vi "Main.vi"(11 "Module Admin":refnum<class "Delacor_lib_QMH_Module Admin.lvclass">) -> ()   [LabVIEW 2021, in "AS-Configuration.lvlib"]
doc: "This template is based off of the Queued Message Handler design pattern and the Queued Message Handler project template that ships with LabVIEW.\n\nThe main difference is that the queue is private to this module and communication between modules is performed via Broadcast and Request events.\n\nRequest events are wrapped in public API methods and are handled in the Event Handling Loop (EHL) of this VI. Any module can register for Broadcast events sent by this module. The EHL generates messages based on user interface actions.\n\nThe Message Handling Loop (MHL) processes messages generated by the EHL, or by other messages. The messages are string values, so new messages can be added easily to the Message Cases case structure in the MHL. Each message cluster can also provide an optional value for Message Data, which is a variant that can be converted to whatever message-specific data is required.\n_____\nBased on DQMH Project Template 7.0.1.1316."
uses:
  AS-Configuration.lvlib
  <vilib>/Delacor/Delacor QMH/Libraries/Module Admin_class/Delacor_lib_QMH_Module Admin.lvclass
  Module Data--cluster.ctl
  Configuration/DO Channel's.ctl
  <vilib>/Wovalab/Utilities/Helper Loop Periodic Timing/Helper Loop Periodic Timing.lvclass/Helper Loop Periodic Timing.ctl
  <vilib>/Delacor/Delacor QMH/Libraries/Message Queue_class/Delacor_lib_QMH_Message Queue.lvclass/Delacor_lib_QMH_Message Queue.ctl
  Stop Argument--cluster.ctl
  <vilib>/Delacor/Delacor QMH/Libraries/Module Admin_class/Delacor_lib_QMH_Module Admin.lvclass/Delacor_lib_QMH_Module Admin.ctl
  <vilib>/Utility/miscctls.llb/LVPointTypeDef.ctl
  Host-Control's/DTT Test folder Name's.ctl
  <vilib>/Delacor/Delacor QMH/Libraries/Message Queue_class/Delacor_lib_QMH_Enqueue Message (Single).vi
  <vilib>/Delacor/Delacor QMH/Libraries/Module Admin_class/Delacor_lib_QMH_Get External Launch.vi
  <vilib>/Wovalab/Utilities/Helper Loop Periodic Timing/U32 Max Value--constant.vi
  <vilib>/Wovalab/Utilities/Helper Loop Periodic Timing/Update Last Execution Time.vi
  <vilib>/Utility/traverseref.llb/TRef Get All FP References.vi
  <vilib>/Utility/traverseref.llb/Get GObject Label.vi
  <vilib>/Utility/xml.llb/Read From XML File.vi
  <vilib>/Utility/xml.llb/Read From XML File(string).vi
  <vilib>/Utility/xml.llb/Write to XML File.vi
  <vilib>/Utility/xml.llb/Write to XML File(string).vi
  <vilib>/Wovalab/Utilities/Helper Loop Periodic Timing/Helper Loop Periodic Timing.lvclass
  <vilib>/Delacor/Delacor QMH/Libraries/Message Queue_class/Delacor_lib_QMH_Message Queue.lvclass
  Main-Module/Host Main.lvlib
  <userlib>/_OpenG.lib/appcontrol/appcontrol.llb/openg_application_control.lvlib
  Configuration/Configuration.lvlib
panel:
  out "Refnum OK?":bool
  out "Given File Name":string
  out "Hw Config File":string caption="Hardware Config File Name"
  in  "New":bool
  in  "Open":bool
  in  "Save":bool
  in  "Table":T1(array[cluster]) {"End Time (S)" min=0.0 max=60.0 step=1.0; "Start Time" min=0.0 max=60.0 step=1.0}
  out "AS-File Name":string caption="Auto-Sequence File Name"
  out "error out":errorcluster
  out "Status":string
  in  "Simulate MHL Error":bool
  in  "Simulate EHL Error":bool
  # "IIT M Drop Tower Test System"
  # "Auto-Sequence Configuration"
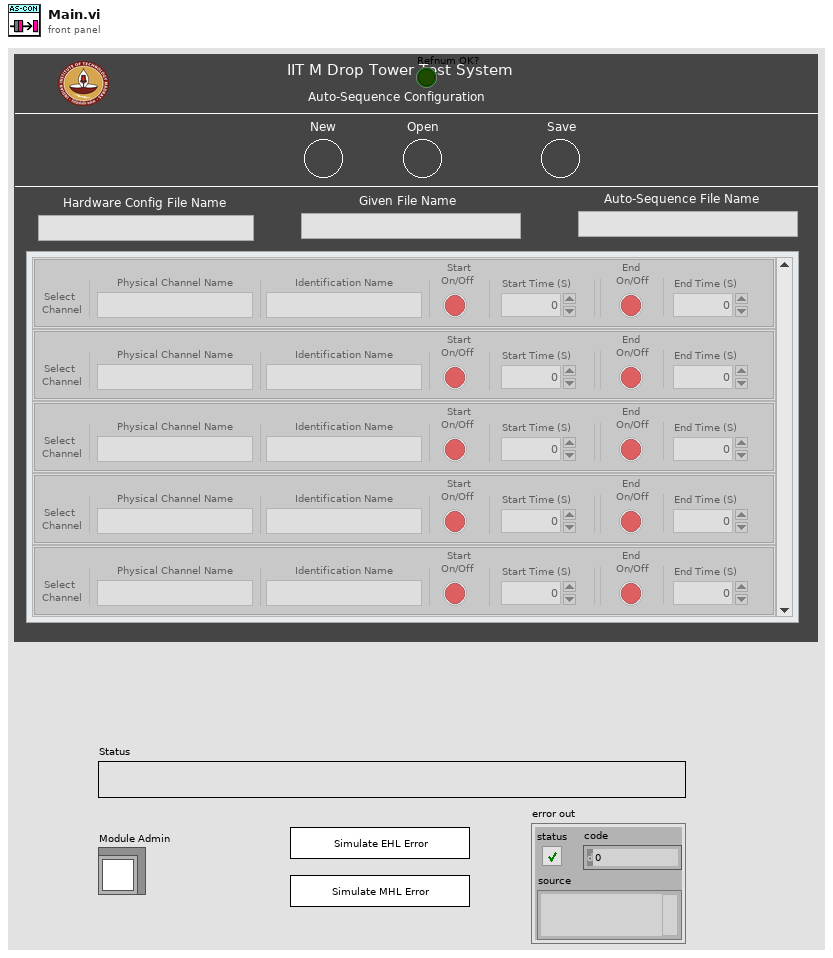
[diagram p1: front panel]
types:
  T1 = cluster{"Select Channel":bool, "Physical Channel Name":string, "Identification Name":string, "  Start\nOn/Off":bool, "Start Time":dbl, "  End\nOn/Off":bool, "End Time (S)":dbl}[]
  T2 = typedef "AS-Configuration.lvlib/Request Events--cluster.ctl" = cluster{"Stop Module":refnum<user-event>, "Show Panel":refnum<user-event>, "Hide Panel":refnum<user-event>, "Get Module Execution Status":refnum<user-event>, "Show Diagram":refnum<user-event>}
  T3 = typedef "AS-Configuration.lvlib/Module Data--cluster.ctl" = cluster{"Status":string, "DO-DI Channel's":T4, "This VI":refnum<vi>, "HW Config File Name":string, "Given File Name":string, "AS-Folder Path":path, "GUI Info's":cluster{"All Object Ref":refnum<vi>[], "All Object Label":string[]}}
  T4 = typedef "Configuration.lvlib/DO Channel's.ctl" = cluster{"Channel Name":string, "Identification Name":string, "Data":u8[], "Enabled?":bool}[]
  T5 = enum32{"invalid lock state", "Not Locked", "Locked (No Password)", "Password-protected"}
  T6 = typedef "AS-Configuration.lvlib/Stop Argument--cluster.ctl" = cluster{"Origin":string, "Exit via Stop Module Req?":bool, "Wait for Module to stop?":bool}
  T7 = typedef "LVPointTypeDef.ctl" = cluster{"Horizontal":i16, "Vertical":i16}
  T8 = enum32{"Invalid", "Standard", "Closed", "Hidden", "Minimized", "Maximized"}
  T9 = typedef "DTT Test folder Name's.ctl" = enum16{"Event Log", "Auto Sequence Configuration", "Channel Configuration's"}
  T10 = cluster{"Select Channel":bool, "Physical Channel Name":string, "Identification Name":string, "  Start\nOn/Off":bool, "Start Time":dbl, "  End\nOn/Off":bool, "End Time (S)":dbl}
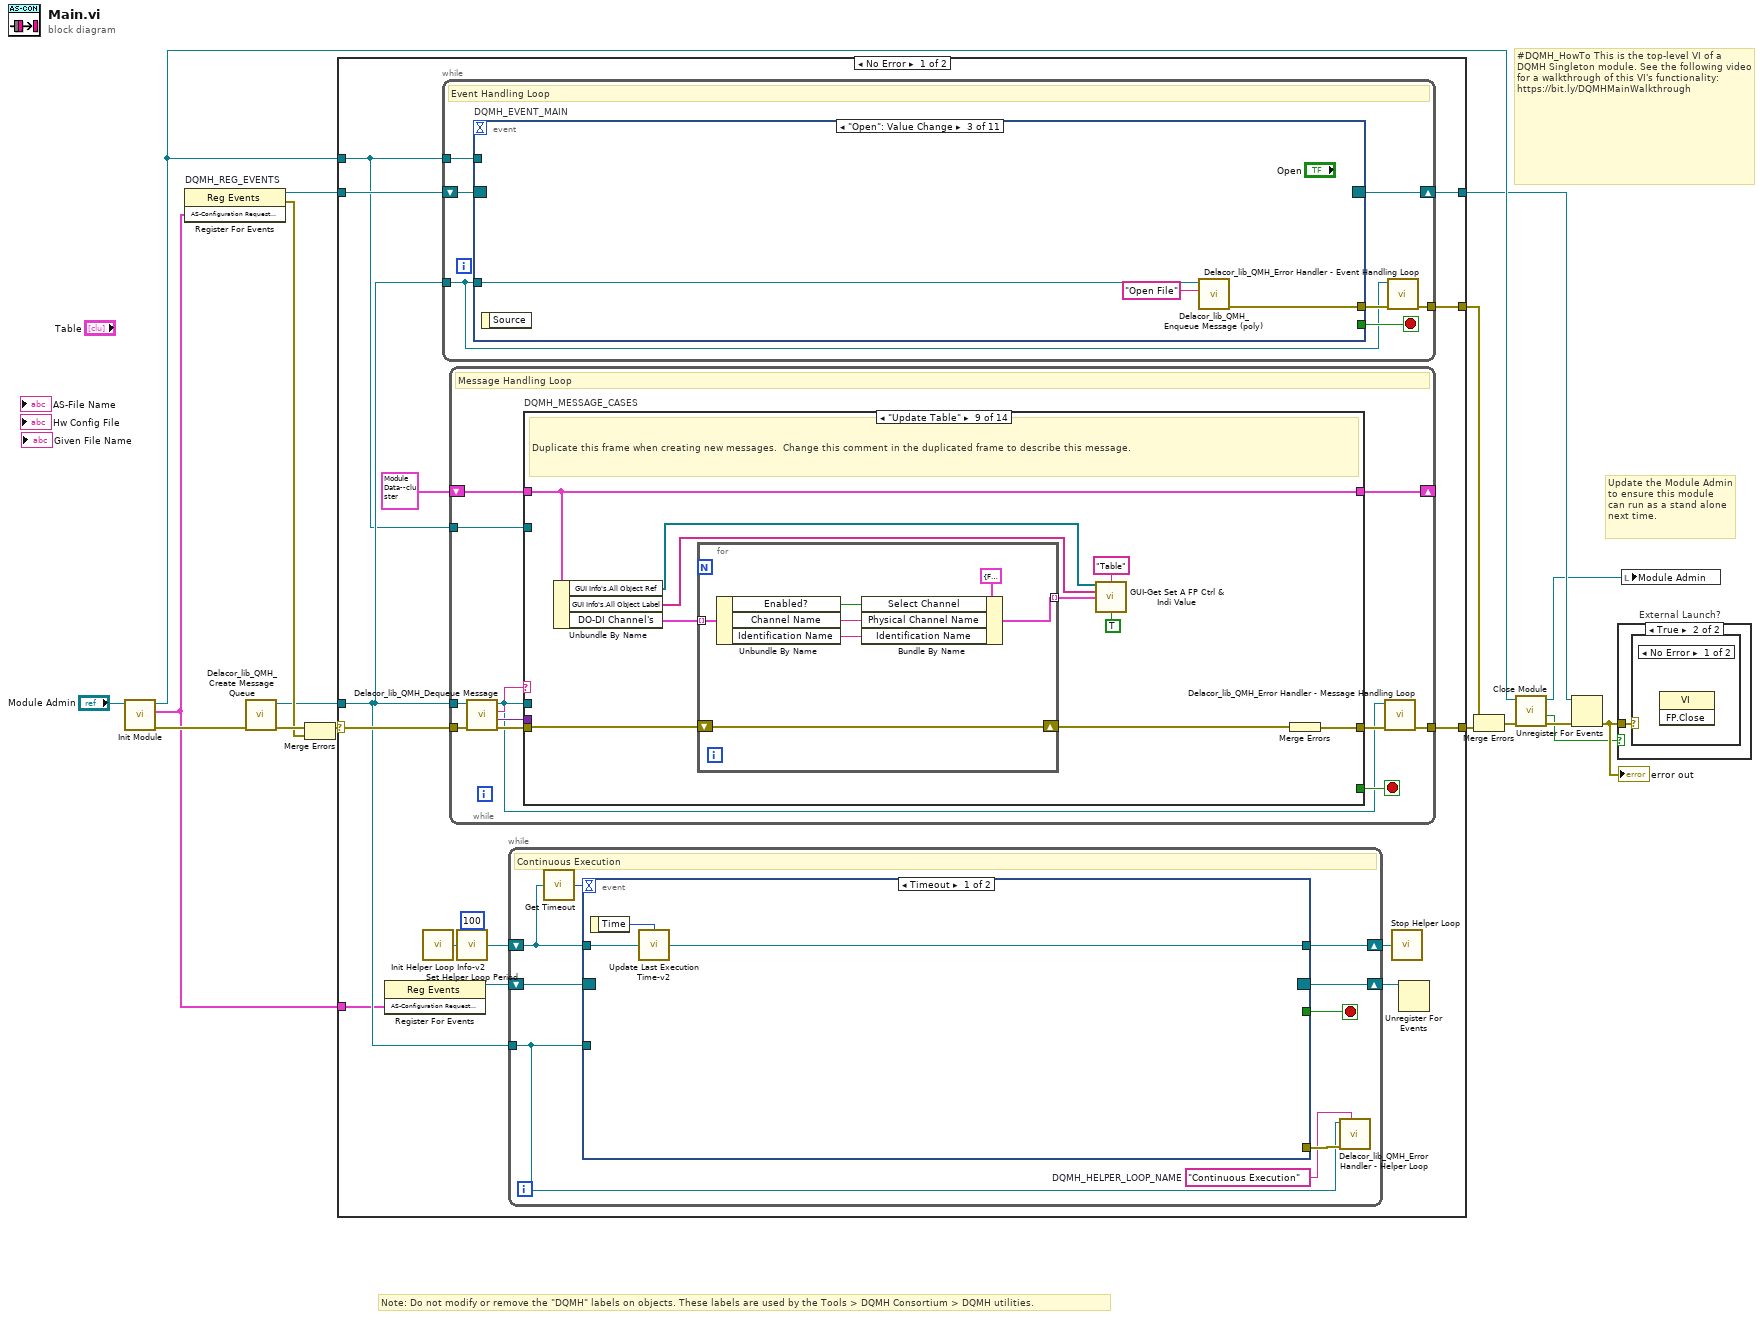
[diagram p0: block diagram]
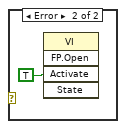
[diagram p3: hidden frame]
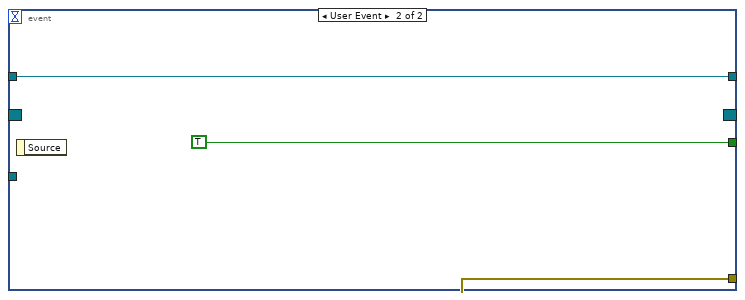
[diagram p4: hidden frame]
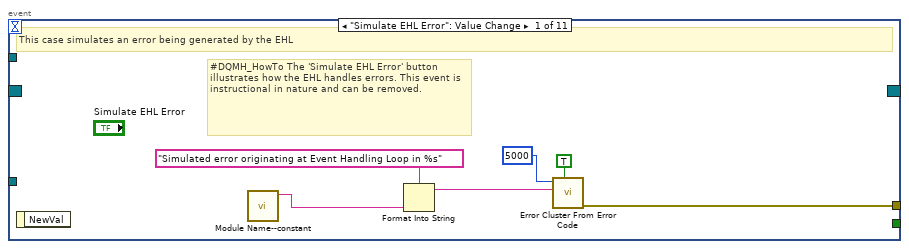
[diagram p5: hidden frame]
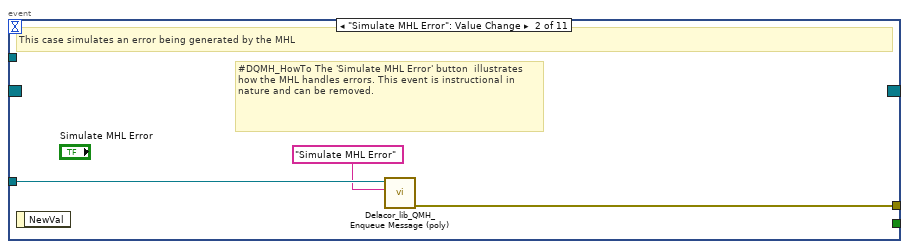
[diagram p6: hidden frame]
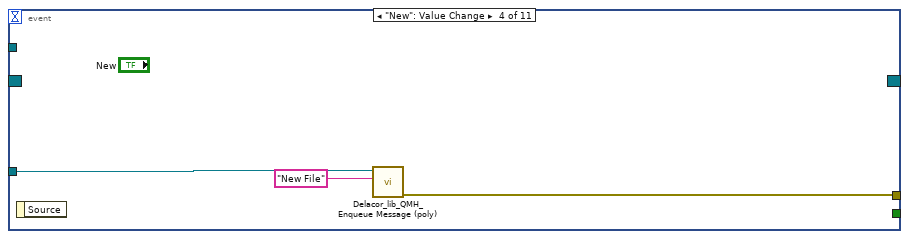
[diagram p7: hidden frame]
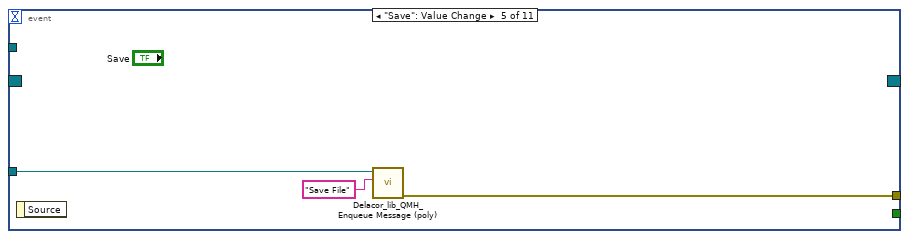
[diagram p8: hidden frame]
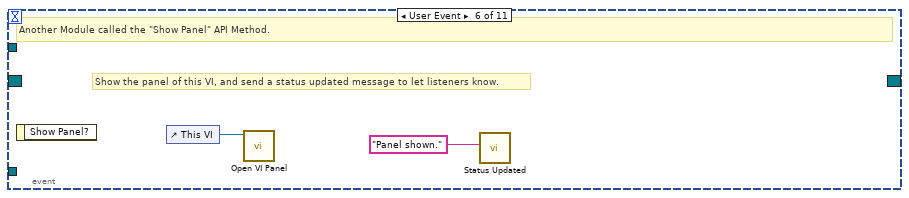
[diagram p9: hidden frame]
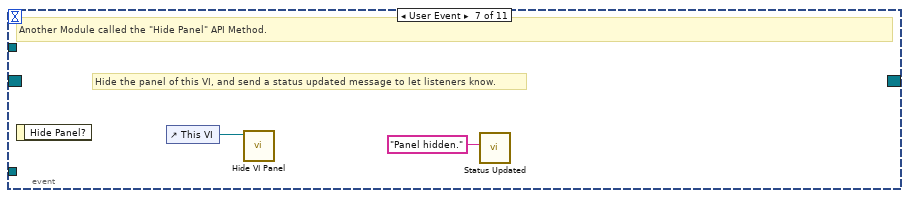
[diagram p10: hidden frame]
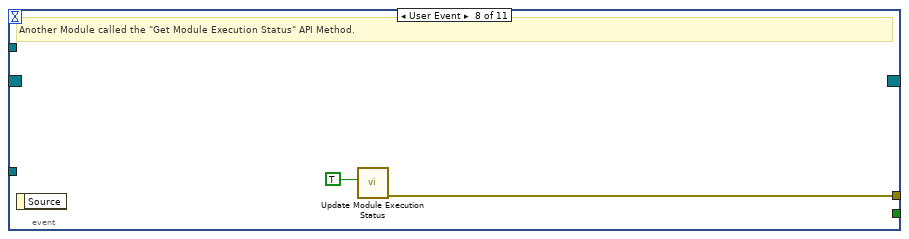
[diagram p11: hidden frame]
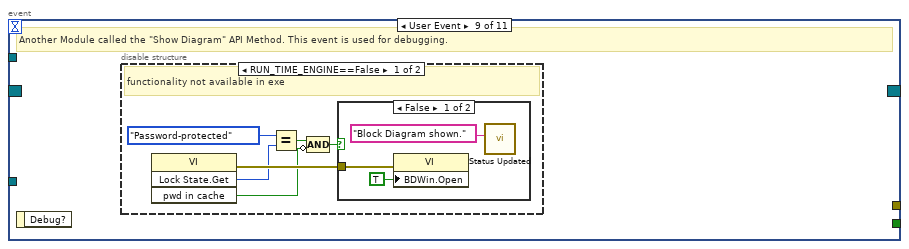
[diagram p12: hidden frame]
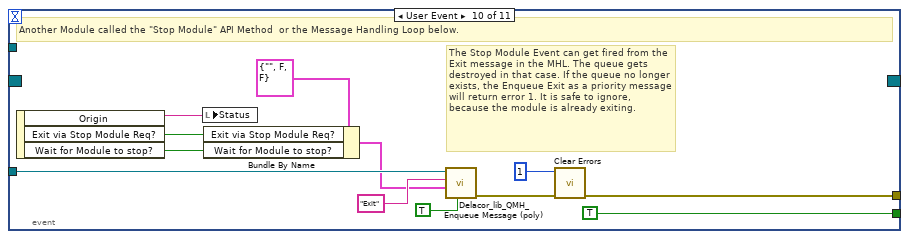
[diagram p15: hidden frame]
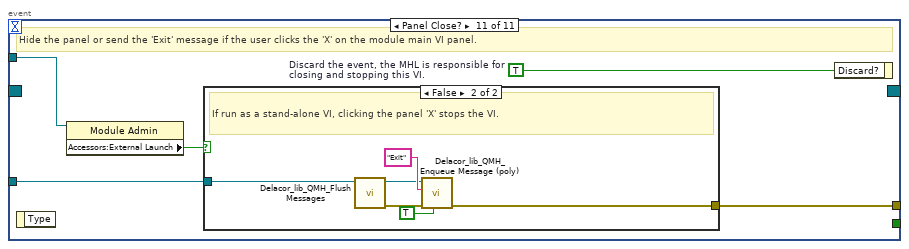
[diagram p16: hidden frame]
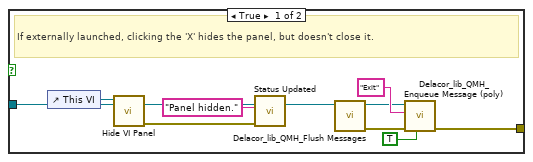
[diagram p17: hidden frame]
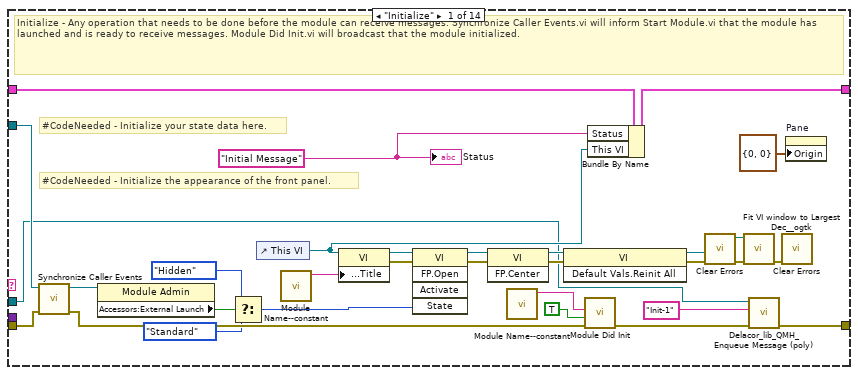
[diagram p18: hidden frame]
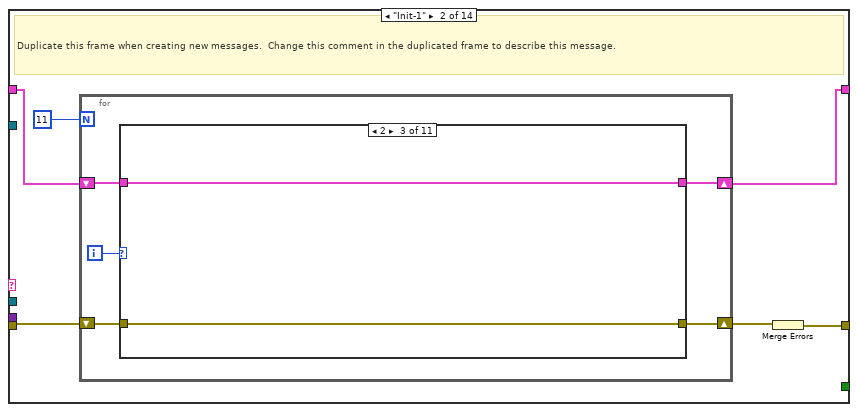
[diagram p19: hidden frame]
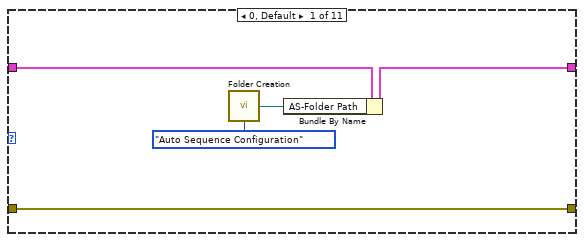
[diagram p20: hidden frame]
diagram:
  # "#DQMH_HowTo This is the top-level VI of a DQMH Singleton module. See the following video for a walkthrough of this VI's functionality: https://bit.ly/DQMHMainWalkthrough"
  # "Note: Do not modify or remove the \"DQMH\" labels on objects. These labels are used by the Tools > DQMH Consortium > DQMH utilities."
  # "Update the Module Admin to ensure this module can run as a stand alone next time."
  n1 = call "Init Module.vi"("Singleton Module Admin in"="Module Admin") -> ("error out"=w16:errorcluster, "AS-Configuration Request Events"=w1:T2, "Singleton Module Admin out"=w8:refnum<class "Delacor_lib_QMH_Module Admin.lvclass">)  [unwired: 8 in]
  n2 = register-events "DQMH_REG_EVENTS"(w1) -> (reference out=w6:refnum<event-registration>, error out=w9:errorcluster)  [unwired: 2 in]
  n3 = call <vilib>:"Delacor_lib_QMH_Create Message Queue.vi"("error in"=w16) -> ("error out"=w11:errorcluster, "Message Queue"=w5:refnum<class "Delacor_lib_QMH_Message Queue.lvclass">)  [unwired: 9 in]
  n4 = Merge Errors(w11, w9) -> (w10:errorcluster)
  n5 = case shown="No Error" w10 {
    selector: w10 -> [w30 w400]
    tunnel: [w32 w399] -> w17
    tunnel: [w29 w398] -> w7
    tunnel: w6 -> [w27 w398]
    tunnel: w5 -> [w26 w393]
    tunnel: [w31 _] -> w14
    tunnel: w8 -> [w25 w394]
    tunnel: w1 -> [w24 _]
    frame No Error {
      n6 = register-events ("DQMH_HELPER_REGFOREVENTS")(w24) -> (reference out=w22:refnum<event-registration>)  [unwired: 2 in, 1 out]
      n7 = call <vilib>:"Init Helper Loop Info-v2.vi"() -> ("Helper Loop Periodic Timing"=w20:refnum<class "Helper Loop Periodic Timing.lvclass">)  [unwired: 1 in]
      n8 = while {
        tunnel: w26 -> [w48]
        shift-right: [w51] -> w29
        shift-left: w27 -> [w52]
        tunnel: [w53] -> w31
        tunnel: w25 -> [w49]
        stop <- w50 stop-if-true
        # "Event Handling Loop"
        n9 = event "DQMH_EVENT_MAIN" shown="[2] \"Open\": Value Change" {
          selector: w52 -> [_ _ _ _ _ _ _ _ _ _ _]
          dyn-events: [_ _ _ _ _ _ _ _ _ _ _] -> w51
          timeout: _ -> [_ _ _ _ _ _ _ _ _ _ _]
          tunnel: [_ _ _ _ _ _ _ _ _ TRUE ("Discard?") _] -> w50
          tunnel: w48 -> [_ w62 w65 w68 w71 _ _ _ _ w95 w102]
          tunnel: [w60 w63 w66 w67 w70 _ _ w78 _ w98 w104] -> w54
          tunnel: w49 -> [_ _ _ _ _ _ _ _ _ _ w101]
          event "Simulate EHL Error": Value Change {
            # "#DQMH_HowTo The 'Simulate EHL Error' button  illustrates how the EHL handles errors. This event is instructional in nature and can be removed."
            # "This case simulates an error being generated by the EHL"
            n10 = event-data() -> ()  [unwired: 1 in, 1 out]
            n11 = call "Module Name--constant.vi"() -> ("Module Name"=w57:string)  [unwired: 11 in]
            n12 = Format Into String(format string="Simulated error originating at Event Handling Loop in %s", w57) -> (resulting string=w58:string)  [unwired: 2 in, 1 out]
            n13 = call <vilib>:"Error Cluster From Error Code.vi"("show call chain? (False)"=TRUE, "error message (\"\")"=w58, "error code (0)"=5000) -> ("error out"=w60:errorcluster)  [unwired: 6 in]
          }
          event "Simulate MHL Error": Value Change {
            # "#DQMH_HowTo The 'Simulate MHL Error' button  illustrates how the MHL handles errors. This event is instructional in nature and can be removed."
            # "This case simulates an error being generated by the MHL"
            n14 = event-data() -> ()  [unwired: 1 in, 1 out]
            n15 = call-poly <vilib>:"Delacor_lib_QMH_Enqueue Message (poly).vi"("Message"="Simulate MHL Error", "Message Queue in"=w62) -> ("error out"=w63:errorcluster)  [unwired: 8 in, 1 out]
          }
          event "Open": Value Change {
            n16 = event-data() -> ()  [unwired: 1 in, 1 out]
            n17 = call-poly <vilib>:"Delacor_lib_QMH_Enqueue Message (poly).vi"("Message"="Open File", "Message Queue in"=w65) -> ("error out"=w66:errorcluster)  [unwired: 8 in, 1 out]
          }
          event "New": Value Change {
            n18 = event-data() -> ()  [unwired: 1 in, 1 out]
            n19 = call-poly <vilib>:"Delacor_lib_QMH_Enqueue Message (poly).vi"("Message"="New File", "Message Queue in"=w68) -> ("error out"=w67:errorcluster)  [unwired: 8 in, 1 out]
          }
          event "Save": Value Change {
            n20 = event-data() -> ()  [unwired: 1 in, 1 out]
            n21 = call-poly <vilib>:"Delacor_lib_QMH_Enqueue Message (poly).vi"("Message"="Save File", "Message Queue in"=w71) -> ("error out"=w70:errorcluster)  [unwired: 8 in, 1 out]
          }
          event User Event {
            # "Show the panel of this VI, and send a status updated message to let listeners know."
            # "Another Module called the \"Show Panel\" API Method."
            n22 = event-data() -> ()  [unwired: 1 in, 1 out]
            n23 = control-ref of="This VI"() -> (w74:refnum<vi>)
            n24 = call "Open VI Panel.vi"("VI"=w74) -> ()  [unwired: 10 in, 1 out]
            n25 = call "Status Updated.vi"("Status"="Panel shown." ("format string")) -> ()  [unwired: 10 in, 1 out]
          }
          event User Event {
            # "Hide the panel of this VI, and send a status updated message to let listeners know."
            # "Another Module called the \"Hide Panel\" API Method."
            n26 = event-data() -> ()  [unwired: 1 in, 1 out]
            n27 = control-ref of="This VI"() -> (w76:refnum<vi>)
            n28 = call "Hide VI Panel.vi"("VI"=w76) -> ()  [unwired: 10 in, 1 out]
            n29 = call "Status Updated.vi"("Status"="Panel hidden." ("format string")) -> ()  [unwired: 10 in, 1 out]
          }
          event User Event {
            # "Another Module called the \"Get Module Execution Status\" API Method."
            n30 = event-data() -> ()  [unwired: 1 in, 1 out]
            n31 = call "Update Module Execution Status.vi"("Running?"=TRUE) -> ("error out"=w78:errorcluster)  [unwired: 10 in]
          }
          event User Event {
            # "Another Module called the \"Show Diagram\" API Method. This event is used for debugging."
            n32 = event-data() -> ()  [unwired: 1 in, 1 out]
            n33 = disable-structure shown="RUN_TIME_ENGINE==False" {
              frame condition #0 (active) {
                # "functionality not available in exe"
                n34 = invoke on="Invoke Node" class="VI" method="Lock State.Get"() -> (error out=w84:errorcluster, "Get Lock State"=w83:T5, "pwd in cache"=w80:bool)  [unwired: 4 in, 1 out]
                n35 = Equal?(x=T5."Password-protected", y=w83) -> (x = y?=w81:bool)
                n36 = Compound Arithmetic op=AND(w81, invert w80) -> (w79:bool)
                n37 = case shown="False" w79 {
                  tunnel: w84 -> [w87 _]
                  frame False {
                    n38 = property on="Property Node" class="VI"(error in=w87, "BDWin.Open"=TRUE ("Block Diagram Window:Open")) -> ()  [unwired: 1 in, 2 out]
                    n39 = call "Status Updated.vi"("Status"="Block Diagram shown." ("format string")) -> ()  [unwired: 10 in, 1 out]
                  }
                  frame True {
                    # "Password-protected VI, and the password is not in the cache. Do not show the diagram."
                  }
                }
              }
              frame condition #1 {
              }
            }
          }
          event User Event {
            # "The Stop Module Event can get fired from the Exit message in the MHL. The queue gets destroyed in that case. If the queue no longer exists, the Enqueue Exit as a priority message will return error 1. It is safe to ignore, because the module is already exiting."
            # "Another Module called the \"Stop Module\" API Method  or the Message Handling Loop below."
            n40 = event-data() -> ("Origin"=w94:string, "Exit via Stop Module Req?"=w90:bool, "Wait for Module to stop?"=w89:bool)  [unwired: 1 in]
            n41 = local write "Status"(w94) -> ()
            n42 = Bundle By Name(cluster=T6 {"Origin"="", "Exit via Stop Module Req?"=FALSE, "Wait for Module to stop?"=FALSE} ("Stop Argument"), "Exit via Stop Module Req?"=w90, "Wait for Module to stop?"=w89) -> (w88:T6)
            n43 = call-poly <vilib>:"Delacor_lib_QMH_Enqueue Message (poly).vi"("Priority Message? (F)"=TRUE, "Message Data"=w88, "Message"="Exit", "Message Queue in"=w95) -> ("error out"=w99:errorcluster)  [unwired: 6 in, 1 out]
            n44 = call <vilib>:"Clear Errors.vi"("error in (no error)"=w99, "specific error code to clear (0: all)"=1) -> ("error out"=w98:errorcluster)  [unwired: 4 in, 1 out]
          }
          event Panel Close? {
            w103 = TRUE  # Discard the event, the MHL is responsible for closing and stopping this VI.
            # "Hide the panel or send the 'Exit' message if the user clicks the 'X' on the module main VI panel."
            n45 = event-data() -> ()  [unwired: 1 in, 1 out]
            n46 = property on="Property Node" class="Module Admin"(reference=w101) -> ("Accessors:External Launch"=w100:bool)  [unwired: 1 in, 2 out]
            n47 = case shown="False" w100 {
              tunnel: w102 -> [w107 w116]
              tunnel: [w108 w119] -> w104
              frame True {
                # "If externally launched, clicking the 'X' hides the panel, but doesn't close it."
                n48 = control-ref of="This VI"() -> (w113:refnum<vi>)
                n49 = call "Hide VI Panel.vi"("VI"=w113) -> ("error out"=w111:errorcluster)  [unwired: 10 in]
                n50 = call "Status Updated.vi"("error in"=w111, "Status"="Panel hidden." ("format string")) -> ()  [unwired: 9 in, 1 out]
                n51 = call-dynamic "Delacor_lib_QMH_Flush Messages.vi"("Message Queue in"=w107) -> ("error out"=w105:errorcluster, "Message Queue out"=w106:refnum<class "Delacor_lib_QMH_Message Queue.lvclass">)  [unwired: 7 in, 2 out]
                n52 = call-poly <vilib>:"Delacor_lib_QMH_Enqueue Message (poly).vi"("Priority Message? (F)"=TRUE, "error in"=w105, "Message"="Exit", "Message Queue in"=w106) -> ("error out"=w108:errorcluster)  [unwired: 6 in, 1 out]
              }
              frame False {
                # "If run as a stand-alone VI, clicking the panel 'X' stops the VI."
                n53 = call-dynamic "Delacor_lib_QMH_Flush Messages.vi"("Message Queue in"=w116) -> ("error out"=w114:errorcluster, "Message Queue out"=w115:refnum<class "Delacor_lib_QMH_Message Queue.lvclass">)  [unwired: 7 in, 2 out]
                n54 = call-poly <vilib>:"Delacor_lib_QMH_Enqueue Message (poly).vi"("Priority Message? (F)"=TRUE, "error in"=w114, "Message"="Exit", "Message Queue in"=w115) -> ("error out"=w119:errorcluster)  [unwired: 6 in, 1 out]
              }
            }
            n55 = event-data ("Event Filter Node")("Discard?"=w103) -> ()  [unwired: 1 in, 1 out]
          }
        }
        n56 = call-dynamic "Delacor_lib_QMH_Error Handler - Event Handling Loop.vi"("error in"=w54, "Message Queue in"=w48) -> ("dup error in"=w53:errorcluster)  [unwired: 8 in, 1 out]
      }
      n57 = while {
        tunnel: w26 -> [w120]
        shift-right: [w128] -> _
        shift-left: T3 {"Status"="", "DO-DI Channel's"=[], "This VI"=refnum, "HW Config File Name"="", "Given File Name"="", "AS-Folder Path"=path "", "GUI Info's"={"All Object Ref"=[], "All Object Label"=[]}} ("Data Cluster") -> [w129]
        tunnel: w30 -> [w131]
        tunnel: [w123] -> w32
        tunnel: w25 -> [w124]
        stop <- w127 stop-if-true
        # "Message Handling Loop"
        n58 = call-dynamic "Delacor_lib_QMH_Dequeue Message.vi"("error in"=w131, "Message Queue in"=w120) -> ("error out"=w130:errorcluster, "Message Data"=w125:variant, "Message"=w126:string, "Message Queue out"=w121:refnum<class "Delacor_lib_QMH_Message Queue.lvclass">)  [unwired: 6 in]
        n59 = case "DQMH_MESSAGE_CASES" shown="\"Update Table\"" w126 {
          selector: w126 -> [_ _ _ _ _ _ _ _ _ _ _ _ _ w388]
          tunnel: w121 -> [w135 _ _ _ w211 _ _ _ _ _ _ w354 w376 _]
          tunnel: w130 -> [w159 w165 w203 w205 w209 w249 w301 w322 w328 w341 w350 w361 w382 w391]
          tunnel: [w133 w167 w203 w205 w214 w246 w303 w321 w332 w341 w349 w357 w377 w392] -> w122
          tunnel: w129 -> [w150 w164 w202 w204 w213 w241 w302 w320 w331 w340 w347 w356 w375 w389]
          tunnel: [w149 w163 w202 w204 w212 w242 w302 w320 w331 w340 w347 w356 w375 w389] -> w128
          tunnel: [_ _ _ _ _ _ _ _ _ _ _ _ w374 _] -> w127
          tunnel: w125 -> [_ _ _ _ _ _ _ _ _ _ _ w355 w373 _]
          tunnel: w124 -> [w151 _ _ _ _ _ _ _ _ _ _ w353 w368 _]
          frame "Initialize" {
            w145 = "Initial Message" ("Initial Message")
            # "#CodeNeeded - Initialize the appearance of the front panel."
            # "#CodeNeeded - Initialize your state data here."
            # "Initialize - Any operation that needs to be done before the module can receive messages. Synchronize Caller Events.vi will inform Start Module.vi that the module has launched and is ready to receive messages. Module Did Init.vi will broadcast that the module initialized."
            n60 = call "Synchronize Caller Events.vi"("error in"=w159, "Singleton Module Admin in"=w151) -> ("error out"=w158:errorcluster, "Singleton Module Admin out"=w146:refnum<class "Delacor_lib_QMH_Module Admin.lvclass">)  [unwired: 8 in]
            n61 = property on="Property Node" class="Module Admin"(reference=w146) -> ("Accessors:External Launch"=w155:bool)  [unwired: 1 in, 2 out]
            n62 = Select(t=T8."Hidden" ("State"), s=w155, f=T8."Standard" ("State")) -> (s? t:f=w152:T8)
            n63 = control-ref of="This VI"() -> (w139:refnum<vi>)
            n64 = call "Module Name--constant.vi"() -> ("Module Name"=w157:string)  [unwired: 11 in]
            n65 = property on="Property Node" class="VI"(reference=w139, "Front Panel.Title"=w157) -> (reference out=w140:refnum<vi>, error out=w161:errorcluster)  [unwired: 1 in]
            n66 = invoke on="Invoke Node" class="VI" method="FP.Open"(reference=w140, error in=w161, "State"=w152) -> (reference out=w156:refnum<vi>, error out=w160:errorcluster)  [unwired: 2 in, 3 out]
            n67 = invoke on="Invoke Node" class="VI" method="FP.Center"(reference=w156, error in=w160) -> (reference out=w142:refnum<vi>, error out=w141:errorcluster)  [unwired: 1 in, 1 out]
            n68 = call "Module Name--constant.vi"() -> ("Module Name"=w147:string)  [unwired: 11 in]
            n69 = invoke class="VI" method="Default Vals.Reinit All"(reference=w142, error in=w141) -> (reference out=w137:refnum<vi>, error out=w138:errorcluster)  [unwired: 1 in, 1 out]
            n70 = call "Module Did Init.vi"("error in"=w158, "Initialized?"=TRUE, "Origin"=w147) -> ("error out"=w134:errorcluster)  [unwired: 8 in]
            n71 = Bundle By Name(cluster=w150, "Status"=w145, "This VI"=w139) -> (w149:T3)
            n72 = call <vilib>:"Clear Errors.vi"("error in (no error)"=w138) -> ("error out"=w136:errorcluster)  [unwired: 5 in, 1 out]
            n73 = call <userlib>:"Fit VI window to Largest Dec__ogtk.vi"("error in (no error)"=w136, "VI Ref (calling VI)"=w137) -> ("error out"=w143:errorcluster)  [unwired: 4 in, 1 out]
            n74 = call-poly <vilib>:"Delacor_lib_QMH_Enqueue Message (poly).vi"("error in"=w134, "Message"="Init-1", "Message Queue in"=w135) -> ("error out"=w133:errorcluster)  [unwired: 7 in, 1 out]
            n75 = call <vilib>:"Clear Errors.vi"("error in (no error)"=w143) -> ()  [unwired: 5 in, 2 out]
            n76 = property on="Pane" class="Pane"("Origin"=T7 {"Horizontal"=0, "Vertical"=0}) -> ()  [unwired: 2 in, 2 out]
            "Status" <- w145
          }
          frame "Init-1" {
            # "Duplicate this frame when creating new messages.  Change this comment in the duplicated frame to describe this message."
            n77 = for {
              N: 11 -> [_]
              shift-right: [w170] -> w166
              shift-left: w165 -> [w169]
              shift-right: [w172] -> w163
              shift-left: w164 -> [w171]
              i -> [w168]
              n78 = case shown="2" w168 {
                tunnel: [w174 w178 w185 w187 w189 w191 w193 w195 w197 w199 w201] -> w172
                tunnel: w171 -> [w175 w181 w185 w187 w189 w191 w193 w195 w197 w199 w201]
                tunnel: [w177 w183 w184 w186 w188 w190 w192 w194 w196 w198 w200] -> w170
                tunnel: w169 -> [w177 w183 w184 w186 w188 w190 w192 w194 w196 w198 w200]
                frame 0, Default {
                  n79 = call "Folder Creation.vi"("Folder Name"=DTT_Test_folder_Name's."Auto Sequence Configuration") -> ("Selected Folder Path Out"=w173:path)  [unwired: 12 in, 2 out]
                  n80 = Bundle By Name(cluster=w175, "AS-Folder Path"=w173) -> (w174:T3)
                }
                frame 1 {
                  n81 = Unbundle By Name(w181) -> ("This VI"=w182:refnum<vi>)
                  n82 = call "GUI-Get all FP Ctrl & Indi Label and Ref.vi"("Respected VI Ref"=w182) -> ("All Object Label"=w179:string[], "All Object Ref"=w180:refnum<vi>[])  [unwired: 9 in]
                  n83 = Bundle By Name(cluster=w181, "GUI Info's.All Object Ref"=w180, "GUI Info's.All Object Label"=w179) -> (w178:T3)
                }
                frame 2 {
                }
                frame 3 {
                }
                frame 4 {
                }
                frame 5 {
                }
                frame 6 {
                }
                frame 7 {
                }
                frame 8 {
                }
                frame 9 {
                }
                frame 10 {
                }
              }
            }
            n84 = Merge Errors(w166) -> (w167:errorcluster)
          }
          frame "---Module Specific---" {
            # "Separator -- The following cases handle messages specific to this Module."
          }
          frame "-----File Operation's-----" {
            # "Separator -- The following cases handle messages specific to this Module."
          }
          frame "New File" {
            # "Duplicate this frame when creating new messages.  Change this comment in the duplicated frame to describe this message."
            n85 = call "Auto Sequence File Name."("error in (no error)"=w209) -> ("File Name"=w207:string, "Ok"=w206:bool, "error out"=w208:errorcluster)  [unwired: 16 in]
            n86 = case shown="True" w206 {
              tunnel: w213 -> [w216 w223]
              tunnel: [w216 w222] -> w212
              tunnel: w211 -> [_ w221]
              tunnel: [w215 w220] -> w210
              tunnel: w208 -> [w215 w219]
              tunnel: w207 -> [_ w218]
              frame False {
              }
              frame True {
                n87 = Empty String/Path?(string/path=w218) -> (empty?=w217:bool)
                n88 = case shown="False" w217 {
                  tunnel: w223 -> [w226 w239]
                  tunnel: [w230 w239] -> w222
                  tunnel: w221 -> [w232 _]
                  tunnel: [w231 w240] -> w220
                  tunnel: w219 -> [w229 w240]
                  tunnel: w218 -> [w225 _]
                  frame False {
                    n89 = Bundle By Name(cluster=w226, "Given File Name"=w225) -> (w224:T3)
                    n90 = call "New AS-File.vi"("Data Cluster In"=w224, "error in"=w229) -> ("error out"=w228:errorcluster, "cancelled"=w227:bool, "Data Cluster Out"=w230:T3)  [unwired: 7 in]
                    n91 = case shown="False" w227 {
                      tunnel: w232 -> [w236 _]
                      tunnel: [w234 w237] -> w231
                      tunnel: w228 -> [w233 w237]
                      frame False {
                        n92 = call-poly <vilib>:"Delacor_lib_QMH_Enqueue Message (poly).vi"("error in"=w233, "Message"="Update Table", "Message Queue in"=w236) -> ("error out"=w234:errorcluster)  [unwired: 7 in, 1 out]
                      }
                      frame True {
                      }
                    }
                  }
                  frame True {
                    n93 = One Button Dialog(message="File Name should not be empty.") -> ()  [unwired: 1 in, 1 out]
                  }
                }
              }
            }
            n94 = Merge Errors(w210) -> (w214:errorcluster)
          }
          frame "Open File" {
            # "Separator -- The following cases handle messages specific to this Module."
            n95 = Unbundle By Name(w241) -> ("GUI Info's.All Object Ref"=w244:refnum<vi>[], "GUI Info's.All Object Label"=w243:string[])
            n96 = call "Folder Creation.vi"("error in"=w249, "Folder Name"=DTT_Test_folder_Name's."Auto Sequence Configuration") -> ("Selected Folder Path Out"=w252:path, "error out"=w251:errorcluster)  [unwired: 11 in, 1 out]
            n97 = call "File Dialog"("start path"=w252, "error in"=w251) -> ("selected path"=w245:path, "cancelled"=w248:bool, "error out"=w247:errorcluster)  [unwired: 10 in, 1 out]
            n98 = case shown="False" w248 {
              tunnel: w247 -> [w255 w280]
              tunnel: [w276 w279] -> w246
              tunnel: w245 -> [w258 _]
              tunnel: w244 -> [w262 _]
              tunnel: w243 -> [w261 _]
              tunnel: [w267 w278] -> w242
              tunnel: w241 -> [w268 w278]
              frame False {
                w257 = T1 [] ("Table")
                n99 = call "XML-Read.vi"("error in (no error)"=w255, "Data"=w257, "XML File Path"=w258) -> ("error out"=w253:errorcluster, "Data Out"=w256:variant, "XML File Path(duplicate)"=w254:path)  [unwired: 6 in]
                n100 = call <vilib>:"Get File Extension.vi"("file"=w254) -> ("filename without extension"=w260:string)  [unwired: 6 in, 4 out]
                n101 = Variant To Data(error in=w253, type=w257, Variant=w256) -> (data=w275:T1, error out=w276:errorcluster)
                n102 = Match Pattern(string=w260, regular expression="_") -> (before substring=w263:string, after substring=w266:string)  [unwired: 1 in, 2 out]
                n103 = call "GUI-Get Set A FP Ctrl & Indi Value.vi"("All Object Ref"=w262, "Label"="Given File Name" ("Label In"), "All Object Label"=w261, "Ctrl Value In"=w263, "Set(F)"=TRUE) -> ()  [unwired: 7 in, 4 out]
                n104 = call "GUI-Get Set A FP Ctrl & Indi Value.vi"("All Object Ref"=w262, "Label"="Table" ("Label In"), "All Object Label"=w261, "Ctrl Value In"=w275, "Set(F)"=TRUE) -> ("Refnum OK?"=→"Refnum OK?":bool)  [unwired: 7 in, 3 out]
                n105 = call "GUI-Get Set A FP Ctrl & Indi Value.vi"("All Object Ref"=w262, "Label"="Hw Config File" ("Label In"), "All Object Label"=w261, "Ctrl Value In"=w266, "Set(F)"=TRUE) -> ()  [unwired: 7 in, 4 out]
                n106 = call "GUI-Get Set A FP Ctrl & Indi Value.vi"("All Object Ref"=w262, "Label"="AS-File Name" ("Label In"), "All Object Label"=w261, "Ctrl Value In"=w260, "Set(F)"=TRUE) -> ()  [unwired: 7 in, 4 out]
                n107 = Bundle By Name(cluster=w268, "Given File Name"=w263, "HW Config File Name"=w266) -> (w267:T3)
              }
              frame True {
                n108 = call <vilib>:"Clear Errors.vi"("error in (no error)"=w280) -> ("error out"=w279:errorcluster)  [unwired: 5 in, 1 out]
              }
            }
          }
          frame "Save File" {
            # "Duplicate this frame when creating new messages.  Change this comment in the duplicated frame to describe this message."
            n109 = Unbundle By Name(w302) -> ("AS-Folder Path"=w299:path, "Given File Name"=w298:string, "HW Config File Name"=w297:string, "GUI Info's.All Object Ref"=w288:refnum<vi>[], "GUI Info's.All Object Label"=w286:string[])
            n110 = call "GUI-Get Set A FP Ctrl & Indi Value.vi"("All Object Ref"=w288, "Label"="Table" ("Label In"), "All Object Label"=w286) -> ("Ctrl Value Out"=w289:variant)  [unwired: 9 in, 3 out]
            n111 = Variant To Data(error in=w301, type=T1 [] ("Table"), Variant=w289) -> (data=w283:T1, error out=w281:errorcluster)
            n112 = for {
              tunnel: [w307] -> w284 mode=indexing if=w304
              tunnel: w283 -> [w307] mode=indexing
              shift-right: [w308] -> w282
              shift-left: w281 -> [w308]
              n113 = Unbundle By Name(w307) -> ("Physical Channel Name"=w306:string)
              n114 = Empty String/Path?(string/path=w306) -> (empty?=w305:bool)
              n115 = Not(x=w305) -> (.not. x?=w304:bool)
            }
            n116 = Empty String/Path?(string/path=w299) -> (empty?=w296:bool)
            n117 = Empty String/Path?(string/path=w297) -> (empty?=w294:bool)
            n118 = Empty String/Path?(string/path=w298) -> (empty?=w295:bool)
            n119 = Not(x=w296) -> (.not. x?=w293:bool)
            n120 = Not(x=w295) -> (.not. x?=w292:bool)
            n121 = Not(x=w294) -> (.not. x?=w291:bool)
            n122 = Compound Arithmetic op=AND(w293, w292, w291) -> (w290:bool)
            n123 = case shown="True" w290 {
              tunnel: [w309 w310] -> w300
              tunnel: w299 -> [_ w317]
              tunnel: w298 -> [_ w316]
              tunnel: w297 -> [_ w315]
              tunnel: w282 -> [w309 w311]
              tunnel: w284 -> [_ w313]
              frame False {
              }
              frame True {
                n124 = Concatenate Strings(w316, "_", w315, ".xml" ("string")) -> (w314:string)
                n125 = Build Path(base path=w317, name or relative path=w314) -> (appended path=w312:path)
                n126 = call "XML-Write.vi"("error in (no error)"=w311, "Data"=w313, "XML File Path"=w312) -> ("error out"=w310:errorcluster)  [unwired: 6 in, 2 out]
              }
            }
            n127 = Merge Errors(w300) -> (w303:errorcluster)
          }
          frame "---Copy This Frame---" {
            # "Duplicate this frame when creating new messages.  Change this comment in the duplicated frame to describe this message."
            n128 = Merge Errors(w322) -> (w321:errorcluster)
          }
          frame "Update Table" {
            # "Duplicate this frame when creating new messages.  Change this comment in the duplicated frame to describe this message."
            n129 = Unbundle By Name(w331) -> ("GUI Info's.All Object Ref"=w324:refnum<vi>[], "GUI Info's.All Object Label"=w323:string[], "DO-DI Channel's"=w330:T4)
            n130 = for {
              tunnel: [w339] -> w325 mode=indexing
              tunnel: w330 -> [w338] mode=indexing
              shift-right: [w333] -> w329
              shift-left: w328 -> [w333]
              n131 = Unbundle By Name(w338) -> ("Enabled?"=w337:bool, "Channel Name"=w336:string, "Identification Name"=w335:string)
              n132 = Bundle By Name(cluster=T10 {"Select Channel"=FALSE, "Physical Channel Name"="", "Identification Name"="", "  Start\nOn/Off"=FALSE, "Start Time"=0.0, "  End\nOn/Off"=FALSE, "End Time (S)"=0.0} ("Cluster"), "Select Channel"=w337, "Physical Channel Name"=w336, "Identification Name"=w335) -> (w339:T10)
            }
            n133 = call "GUI-Get Set A FP Ctrl & Indi Value.vi"("All Object Ref"=w324, "Label"="Table" ("Label In"), "All Object Label"=w323, "Ctrl Value In"=w325, "Set(F)"=TRUE) -> ()  [unwired: 7 in, 4 out]
            n134 = Merge Errors(w329) -> (w332:errorcluster)
          }
          frame "---Exit and Error Handling---" {
            # "Separator - The following cases handle errors and exit messages."
          }
          frame "Simulate MHL Error" {
            # "#DQMH_HowTo The 'Simulate MHL Error' button  illustrates how the MHL handles errors. This event is instructional in nature and can be removed."
            # "Simulate an error occurring at the MHL"
            n135 = call "Module Name--constant.vi"() -> ("Module Name"=w343:string)  [unwired: 11 in]
            n136 = Format Into String(format string="Simulated error originating at Message Handling Loop in %s", w343) -> (resulting string=w344:string)  [unwired: 2 in, 1 out]
            n137 = call <vilib>:"Error Cluster From Error Code.vi"("show call chain? (False)"=TRUE, "error message (\"\")"=w344, "error code (0)"=5001) -> ("error out"=w348:errorcluster)  [unwired: 6 in]
            n138 = Merge Errors(w350, w348) -> (w349:errorcluster)
          }
          frame "Error" {
            # "#CodeRecommended - If the module is running in standalone mode (External Launch = FALSE), this code will pop up an error dialog and call the 'Exit' message if an error occurs. Add more fine-grained error management here."
            # "Error - Check the error message data and respond accordingly. This message is sent by the \"Error Handler\" VIs at the end of each loop in this application."
            n139 = property on="Property Node" class="Module Admin"(reference=w353) -> ("Accessors:External Launch"=w352:bool)  [unwired: 1 in, 2 out]
            n140 = Variant To Data(error in=w361, type=errorcluster {"status"=FALSE, "code"=0, "source"=""} ("error constant"), Variant=w355) -> (data=w351:errorcluster, error out=w359:errorcluster)
            n141 = local write "error out"(w351) -> ()
            n142 = call "Error Reported.vi"("Error"=w351) -> ()  [unwired: 10 in, 1 out]
            n143 = case shown="False" w352 {
              tunnel: [w366 _] -> w358
              tunnel: w354 -> [w364 _]
              tunnel: w351 -> [w365 _]
              frame False {
                n144 = disable-structure shown="Default" {
                  disable-tunnel: w365 -> [w367 _]
                  frame condition #0 (active) {
                    # "If the module is running standalone, then pop up an error dialog and call the \"Exit\" message."
                    n145 = call <vilib>:"Simple Error Handler.vi"("error in (no error)"=w367) -> ()  [unwired: 4 in, 5 out]
                  }
                  frame condition #1 {
                    # "To prevent the Simple Error Handler VI from being loaded (e.g. when deploying to a Real-Time target), add the Conditional Disable Symbol \"DQMH_Disable_SEH\" to your project and set it to TRUE."
                  }
                }
                n146 = call-poly <vilib>:"Delacor_lib_QMH_Enqueue Message (poly).vi"("Priority Message? (F)"=TRUE, "Message"="Exit", "Message Queue in"=w364) -> ("error out"=w366:errorcluster)  [unwired: 7 in, 1 out]
              }
              frame True {
                # "If the module was launched externally, calling the Error Reported broadcast VI is the only action performed by the \"Error\" message. The module's caller can then process the error appropriately."
              }
            }
            n147 = Merge Errors(w359, w358) -> (w357:errorcluster)
          }
          frame "Exit" {
            w372 = 91  # 91: not all Exit messages will have an argument
            w374 = TRUE  # Stop the VI
            # "Release the message queue reference"
            # "#CodeNeeded - Add any required cleanup code here."
            # "Exit - Exit the application."
            n148 = Variant To Data(error in=w382, type=T6 {"Origin"="", "Exit via Stop Module Req?"=FALSE, "Wait for Module to stop?"=FALSE} ("Stop Argument"), Variant=w373) -> (data=w370:T6, error out=w379:errorcluster)
            n149 = call <vilib>:"Clear Errors.vi"("error in (no error)"=w379, "specific error code to clear (0: all)"=w372) -> ("error out"=w381:errorcluster)  [unwired: 4 in, 1 out]
            n150 = control-ref of="This VI"() -> (w369:refnum<vi>)
            n151 = call-dynamic "Delacor_lib_QMH_Release Message Queue.vi"("error in"=w381, "Message Queue"=w376) -> ("error out"=w380:errorcluster)  [unwired: 9 in]
            n152 = call "Handle Exit.vi"("Stop Argument"=w370, "Admin in"=w368, "VI reference"=w369) -> ("error out"=w378:errorcluster)  [unwired: 7 in, 1 out]
            n153 = Merge Errors(w380, w378) -> (w377:errorcluster)
            n154 = call "Error Reported.vi"("Error"=w377) -> ()  [unwired: 10 in, 1 out]
            n155 = call "Show Panel.vi"() -> ()  [unwired: 11 in, 1 out]
          }
          frame Default {
            # "'Default' case only runs if there is a message that isn't defined in any of the other cases.  Output a programming error."
            n156 = call "Module Name--constant.vi"() -> ("Module Name"=w387:string)  [unwired: 11 in]
            n157 = Format Into String(format string="The invalid message string \"%s\" was received in the Message Handling Loop for module \"%s\".", w388, w387) -> (resulting string=w383:string)  [unwired: 2 in, 1 out]
            n158 = call <vilib>:"Error Cluster From Error Code.vi"("show call chain? (False)"=TRUE, "error message (\"\")"=w383, "error code (0)"=1) -> ("error out"=w390:errorcluster)  [unwired: 6 in]
            n159 = Merge Errors(w391, w390) -> (w392:errorcluster)
          }
        }
        n160 = call-dynamic "Delacor_lib_QMH_Error Handler - Message Handling Loop.vi"("error in"=w122, "Message Queue in"=w121) -> ("dup error in"=w123:errorcluster)  [unwired: 8 in, 1 out]
      }
      n161 = call <vilib>:"Set Helper Loop Period.vi"("Period (ms)"=100, "Helper Loop Periodic Timing in"=w20) -> ("Helper Loop Periodic Timing out"=w21:refnum<class "Helper Loop Periodic Timing.lvclass">)  [unwired: 13 in]
      n162 = while "DQMH_HELPER_LOOP" {
        shift-right: [w41] -> w18
        shift-left: w21 -> [w34]
        shift-right: [w39] -> w23
        shift-left: w22 -> [w40]
        tunnel: w26 -> [w36]
        stop <- w38 stop-if-true
        w35 = "Continuous Execution"  # DQMH_HELPER_LOOP_NAME
        # "Continuous Execution"
        n163 = call <vilib>:"Get Timeout.vi"("Helper Loop Periodic Timing"=w34) -> ("Timeout (ms)"=w33:i32)  [unwired: 12 in, 2 out]
        n164 = event "DQMH_HELPER_EVENT_STRUCTURE" shown="[0] Timeout" {
          selector: w40 -> [_ _]
          dyn-events: [_ _] -> w39
          timeout: w33 -> [_ _]
          tunnel: w34 -> [w43 w47]
          tunnel: [w42 w47] -> w41
          tunnel: [_ TRUE] -> w38
          tunnel: [_ errorcluster {"status"=FALSE, "code"=0, "source"=""} ("error constant")] -> w37
          tunnel: w36 -> [_ _]
          event Timeout {
            n165 = event-data() -> ("Time"=w44:u32)  [unwired: 1 in]
            n166 = call <vilib>:"Update Last Execution Time-v2.vi"("Time"=w44, "Helper Loop Periodic Timing in"=w43) -> ("Helper Loop Periodic Timing out"=w42:refnum<class "Helper Loop Periodic Timing.lvclass">)  [unwired: 12 in, 1 out]
          }
          event User Event {
            n167 = event-data() -> ()  [unwired: 1 in, 1 out]
          }
        }
        n168 = call-dynamic "Delacor_lib_QMH_Error Handler - Helper Loop.vi"("Error Debug"=w35, "error in"=w37, "Message Queue in"=w36) -> ()  [unwired: 7 in, 2 out]
      }
      n169 = call <vilib>:"Stop Helper Loop.vi"("Helper Loop Periodic Timing in"=w18) -> ()  [unwired: 1 out]
      n170 = Unregister For Events(event registration refnum=w23) -> ()  [unwired: 1 in, 1 out]
    }
    frame Error {
      # "Synchronize Caller Events.vi will inform Start Module.vi that the module has launched and will let the code calling Start Module.vi register for broadcasts and would permit the caller receive the broadcast that an error occurred at launch time."
      n171 = call-dynamic "Delacor_lib_QMH_Release Message Queue.vi"("error in"=w400, "Message Queue"=w393) -> ("error out"=w399:errorcluster)  [unwired: 9 in]
      n172 = call "Synchronize Caller Events.vi"("Singleton Module Admin in"=w394) -> ("error out"=w401:errorcluster)  [unwired: 9 in, 1 out]
      n173 = call "Module Name--constant.vi"() -> ("Module Name"=w397:string)  [unwired: 11 in]
      n174 = Format Into String(format string="An error occurred during initialization. %s is no longer running.", w397) -> (resulting string=w395:string)  [unwired: 2 in, 1 out]
      n175 = Merge Errors(w399, w401) -> (w402:errorcluster)
      n176 = call "Error Reported.vi"("Additional Information"=w395, "Error"=w402) -> ()  [unwired: 9 in, 1 out]
    }
  }
  n177 = Merge Errors(w14, w17) -> (w13:errorcluster)
  n178 = call "Close Module.vi"("error in"=w13, "Module Admin in"=w8) -> ("error out"=w15:errorcluster, "External Launch"=w2:bool, "Module Admin out"=w3:refnum<class "Delacor_lib_QMH_Module Admin.lvclass">)  [unwired: 7 in]
  n179 = Unregister For Events(event registration refnum=w7, error in=w15) -> (error out=w12:errorcluster)
  "error out" <- w12
  n180 = case "External Launch?" shown="True" w2 {
    tunnel: w12 -> [_ w403]
    frame False {
    }
    frame True {
      n181 = case shown="No Error" w403 {
        frame No Error {
          n182 = invoke on="Invoke Node" class="VI" method="FP.Close"() -> ()  [unwired: 3 in, 3 out]
        }
        frame Error {
          n183 = invoke on="Invoke Node" class="VI" method="FP.Open"("Activate"=TRUE ("Activate?")) -> ()  [unwired: 4 in, 5 out]
        }
      }
    }
  }
  n184 = local write "Module Admin"(w3) -> ()
